vi "Write String.vi"(8 "error in (no error)":errorcluster, 10 "String":string, 11 "StringPayload in":refnum<class "StringPayload.lvclass">) -> (0 "error out":errorcluster, 3 "StringPayload out":refnum<class "StringPayload.lvclass">)   [LabVIEW 2019, in "StringPayload.lvclass"]
uses:
  StringPayload.lvclass
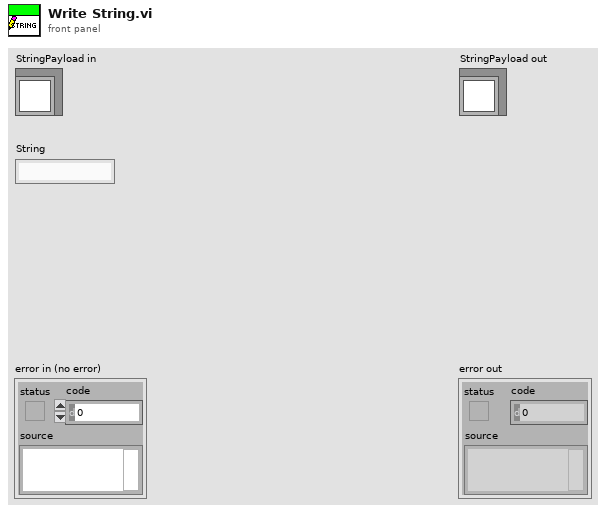
[diagram p1: front panel]
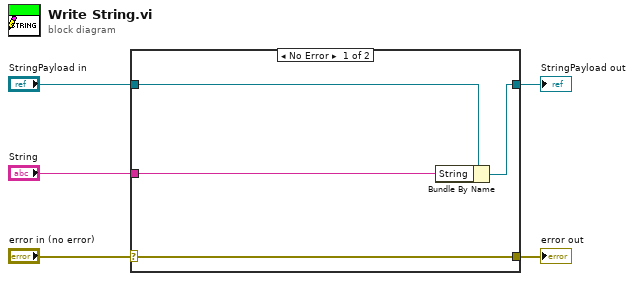
[diagram p0: block diagram]
diagram:
  n1 = case shown="No Error" "error in (no error)" {
    selector: "error in (no error)" -> [w9 w10]
    tunnel: [w9 w10] -> w4
    tunnel: [w7 w11] -> w2
    tunnel: "StringPayload in" -> [w8 w11]
    tunnel: "String" -> [w6 _]
    frame No Error {
      n2 = Bundle By Name(cluster=w8, "String"=w6) -> (w7:refnum<class "StringPayload.lvclass">)
    }
    frame Error {
    }
  }
  "error out" <- w4
  "StringPayload out" <- w2
